vi "HTTP.vi"(6 "Enum":enum16{"close", "post", "get", "init"}(ring), 8 "error in (no error)":errorcluster, 10 "data in":string="http://127.0.0.1:8001/v1/get_data", 11 "url":string="http://127.0.0.1:8001/v1/get_data") -> (0 "error out":errorcluster, 2 "data out":string="http://127.0.0.1:8001/v1/get_data")   [LabVIEW 2014]
uses:
  <vilib>/httpClient/ClientHandle.ctl
  <vilib>/httpClient/POSTBuffer.vi
  <vilib>/httpClient/LabVIEWHTTPClient.lvlib
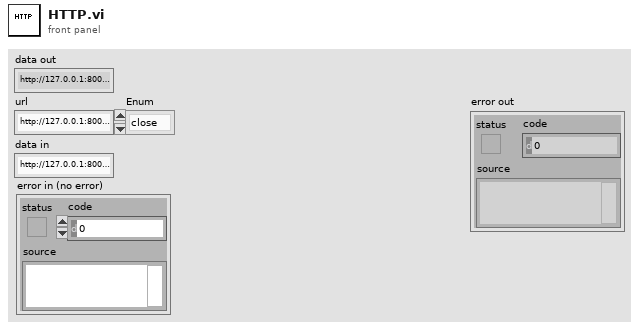
[diagram p1: front panel]
types:
  T1 = typedef "LabVIEWHTTPClient.lvlib/ClientHandle.ctl" = refnum<k1>
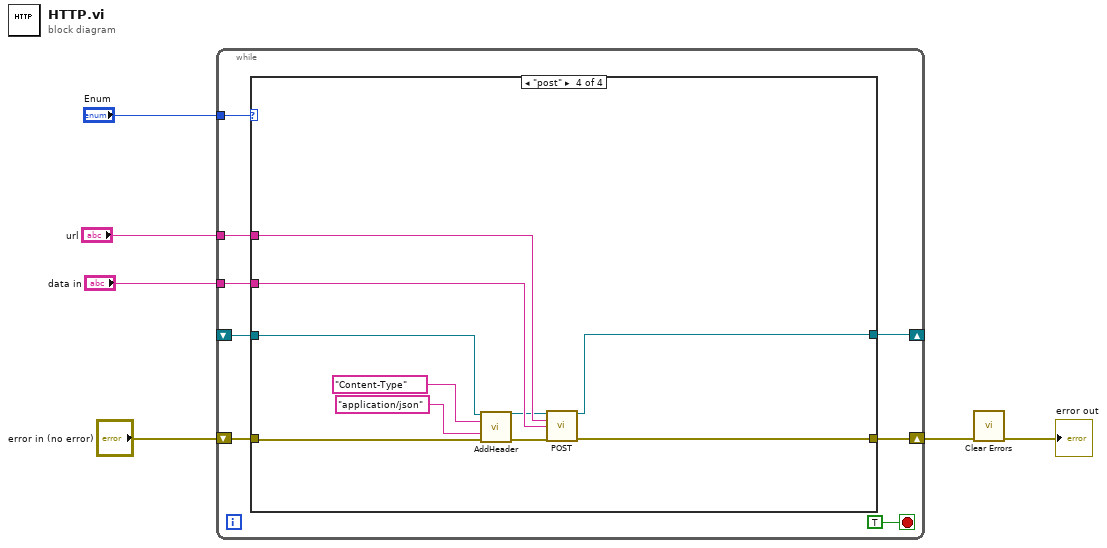
[diagram p0: block diagram]
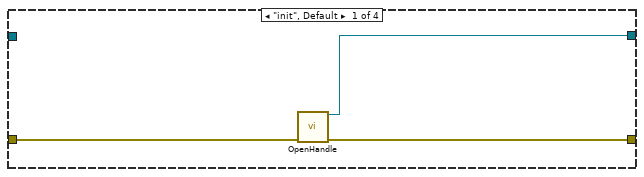
[diagram p2: hidden frame]
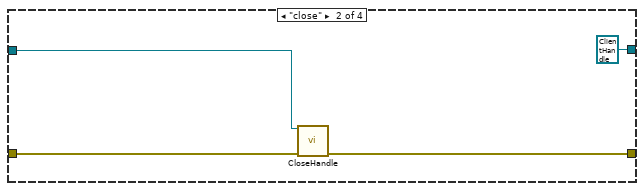
[diagram p3: hidden frame]
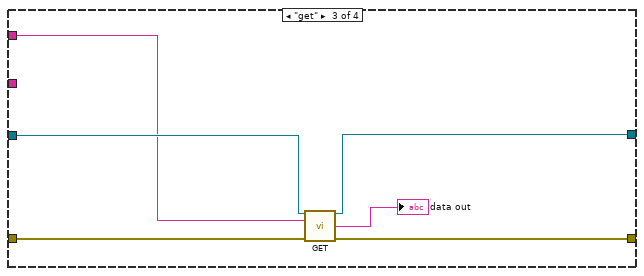
[diagram p4: hidden frame]
diagram:
  n1 = while {
    shift-right: [w13] -> w5
    shift-left: "error in (no error)" -> [w14]
    tunnel: "Enum" -> [w11]
    shift-right: [w10] -> _
    shift-left: _ -> [w7]
    tunnel: "data in" -> [w9]
    tunnel: "url" -> [w8]
    stop <- TRUE stop-if-true
    n2 = case shown="\"post\"" w11 {
      tunnel: w14 -> [w17 w21 w27 w29]
      tunnel: [w16 w20 w26 w37] -> w13
      tunnel: [w15 T1 refnum ("client handle out") w22 w35] -> w10
      tunnel: w9 -> [_ _ _ w34]
      tunnel: w8 -> [_ _ w24 w36]
      tunnel: w7 -> [_ w19 w25 w28]
      frame "init", Default {
        n3 = call <vilib>:"OpenHandle.vi"("error in (no error)"=w17) -> ("client handle out"=w15:T1, "error out"=w16:errorcluster)  [unwired: 13 in]
      }
      frame "close" {
        n4 = call <vilib>:"CloseHandle.vi"("client handle"=w19, "error in (no error)"=w21) -> ("error out"=w20:errorcluster)  [unwired: 13 in]
      }
      frame "get" {
        n5 = call <vilib>:"GET.vi"("client handle"=w25, "url"=w24, "error in (no error)"=w27) -> ("client handle out"=w22:T1, "body"=→"data out":string, "error out"=w26:errorcluster)  [unwired: 9 in, 1 out]
      }
      frame "post" {
        n6 = call <vilib>:"AddHeader.vi"("client handle"=w28, "header"="Content-Type", "value"="application/json", "error in (no error)"=w29) -> ("client handle out"=w31:T1, "error out"=w30:errorcluster)  [unwired: 10 in]
        n7 = call-poly <vilib>:"POST.vi"("client handle"=w31, "url"=w36, "buffer"=w34, "error in (no error)"=w30) -> ("client handle out"=w35:T1, "error out"=w37:errorcluster)  [unwired: 8 in, 2 out]
      }
    }
  }
  n8 = call <vilib>:"Clear Errors.vi"("error in (no error)"=w5) -> ("error out"=→"error out":errorcluster)  [unwired: 5 in, 1 out]
